vi "MGCC_GetLoadCombinations.vi"(8 "List pf critical loads":dbl[](array[numeric]), 9 "List of loads":dbl[](array[numeric]), 11 "MG topology":dbl[][](array[numeric])) -> (0 "crit_index":i32[](array[numeric]), 1 "ValidComb":i32[][](array[numeric]), 2 "Load_Combinations":i32[][](array[numeric]))   [LabVIEW 2016]
uses:
  <vilib>/imath/engines/lvmath2/RunTimeEngine/IndexRead/NIMS M($,S).vi
  <instcachedir>/0/NIMS M($,S)_3E5749BBB62E49528D4765A77F1F6D98.lvgen/NIMS M($,S)_3E5749BBB62E49528D4765A77F1F6D98_000.vi
  <vilib>/imath/engines/lvmath2/RunTimeEngine/BitwiseOperatorToken/NIMS_Bitwise_Operator_Or.vi
  <instcachedir>/0/NIMS_Bitwise_Operator_Or_51E58CBCE6004B7AAA420A8AC17D98D6.lvgen/NIMS_Bitwise_Operator_Or_51E58CBCE6004B7AAA420A8AC17D98D6_001.vi
  <vilib>/imath/engines/lvmath2/RunTimeEngine/VariableToken/Support/NIMS_Vector Boolean Index to I32 Index.vi
  <vilib>/imath/engines/lvmath2/RunTimeEngine/IndexRead/NIMS M(V,$).vi
  <instcachedir>/0/NIMS M(V,$)_21A5155762F74C04AE4EA67BEE0D3EF5.lvgen/NIMS M(V,$)_21A5155762F74C04AE4EA67BEE0D3EF5_004.vi
  <vilib>/imath/engines/lvmath2/RunTimeEngine/ErrorHandling/NIMS_Create Error From Enums.vi
  <vilib>/imath/engines/lvmath2/RunTimeEngine/BuiltInFunctions/findnz/NIMS_[1o]_findnz(GColV).vi
  <instcachedir>/0/NIMS_[1o]_findnz(GColV)_8556557C9365446B906472366DD9B2D8.lvgen/NIMS_[1o]_findnz(GColV)_8556557C9365446B906472366DD9B2D8_000.vi
  <vilib>/imathl/engines/lvmath/Functions/Error Handling/Create Error.vi
  <vilib>/imath/engines/lvmath2/RunTimeEngine/IndexReplace/NIMS M(V,$)=M.vi
  <instcachedir>/0/NIMS M(V,$)=M_4780607DE7B3494DB49F84B9239A732B.lvgen/NIMS M(V,$)=M_4780607DE7B3494DB49F84B9239A732B_003.vi
  <vilib>/imath/engines/lvmath2/RunTimeEngine/BuiltInFunctions/size/NIMS_I32=size(GM,I32).vi
  <instcachedir>/0/NIMS_I32=size(GM,I32)_122058B1B3294FAEA5DC209B92B394E4.lvgen/NIMS_I32=size(GM,I32)_122058B1B3294FAEA5DC209B92B394E4_004.vi
  <vilib>/imath/engines/lvmath2/RunTimeEngine/BuiltInFunctions/length/NIMS_length(GV).vi
  <instcachedir>/0/NIMS_length(GV)_08A3D13377FD4E4B96F5795FBF3698FA.lvgen/NIMS_length(GV)_08A3D13377FD4E4B96F5795FBF3698FA_000.vi
  <vilib>/imath/engines/lvmath2/RunTimeEngine/RangeToken/NIMS_Range_R2 - Integer.vi
  <instcachedir>/0/NIMS_Range_R2 - Integer_89B873E74E6E489885E44F751DD9C6BF.lvgen/NIMS_Range_R2 - Integer_89B873E74E6E489885E44F751DD9C6BF_000.vi
  <vilib>/imath/engines/lvmath2/RunTimeEngine/CommandStatement/MC_CommandStatement_break.vi
  <vilib>/imath/engines/lvmath2/RunTimeEngine/IndexRead/NIMS V(S).vi
  <instcachedir>/0/NIMS V(S)_0488751826AF41519A22953C041130DC.lvgen/NIMS V(S)_0488751826AF41519A22953C041130DC_000.vi
  <vilib>/imath/engines/lvmath2/RunTimeEngine/IndexReplace/NIMS V(V)=M.vi
  <instcachedir>/0/NIMS V(V)=M_7678915A266E4CDB8C8DB8FB3DB4E364.lvgen/NIMS V(V)=M_7678915A266E4CDB8C8DB8FB3DB4E364_001.vi
  <vilib>/imath/engines/lvmath2/RunTimeEngine/VariableToken/NIMS_VariableToken_CondDefinedDefinedByReplace.vi
  <instcachedir>/0/NIMS_VariableToken_CondDefinedDefinedByReplace_D162CFFC24174562A9FEA619A91E1A56.lvgen/NIMS_VariableToken_CondDefinedDefinedByReplace_D162CFFC24174562A9FEA619A91E1A56_003.vi
  <vilib>/imath/engines/lvmath2/RunTimeEngine/BuiltInFunctions/findnz/NIMS_[1o]_findnz(GRowV).vi
  <instcachedir>/0/NIMS_[1o]_findnz(GRowV)_1AF74843B4874134ADE908C0A4A72F3C.lvgen/NIMS_[1o]_findnz(GRowV)_1AF74843B4874134ADE908C0A4A72F3C_000.vi
  <vilib>/imath/engines/lvmath2/RunTimeEngine/IndexReplace/NIMS V(S)=V.vi
  <instcachedir>/0/NIMS V(S)=V_623363232DF04CF88CEE4AC156064DF2.lvgen/NIMS V(S)=V_623363232DF04CF88CEE4AC156064DF2_000.vi
  <instcachedir>/0/NIMS_VariableToken_CondDefinedDefinedByReplace_D162CFFC24174562A9FEA619A91E1A56.lvgen/NIMS_VariableToken_CondDefinedDefinedByReplace_D162CFFC24174562A9FEA619A91E1A56_002.vi
  <vilib>/imath/engines/lvmath2/RunTimeEngine/IndexRead/NIMS M(S,S).vi
  <instcachedir>/0/NIMS M(S,S)_AC51E74150A542F7991B9634C66F3096.lvgen/NIMS M(S,S)_AC51E74150A542F7991B9634C66F3096_000.vi
  <vilib>/imath/engines/lvmath2/RunTimeEngine/IndexReplace/NIMS M(S,S)=S.vi
  <instcachedir>/0/NIMS M(S,S)=S_98E40400474E4398B113AE20298B4F82.lvgen/NIMS M(S,S)=S_98E40400474E4398B113AE20298B4F82_002.vi
  <vilib>/imath/engines/lvmath2/RunTimeSupport/NIMS_Error if Not Equal.vi
  <instcachedir>/0/NIMS_Error if Not Equal_43252A79AD05436189442EC0C5E5AB8A.lvgen/NIMS_Error if Not Equal_43252A79AD05436189442EC0C5E5AB8A_000.vi
  <vilib>/imath/engines/lvmath2/RunTimeEngine/VariableToken/NIMS_VariableToken_CondDefined.vi
  <instcachedir>/0/NIMS_VariableToken_CondDefined_06E9DA95BD4D46A6BA55EC651A891960.lvgen/NIMS_VariableToken_CondDefined_06E9DA95BD4D46A6BA55EC651A891960_009.vi
  <instcachedir>/0/NIMS_I32=size(GM,I32)_122058B1B3294FAEA5DC209B92B394E4.lvgen/NIMS_I32=size(GM,I32)_122058B1B3294FAEA5DC209B92B394E4_005.vi
  <instcachedir>/0/NIMS_VariableToken_CondDefined_06E9DA95BD4D46A6BA55EC651A891960.lvgen/NIMS_VariableToken_CondDefined_06E9DA95BD4D46A6BA55EC651A891960_005.vi
  <vilib>/imath/engines/lvmath2/RunTimeEngine/BuiltInFunctions/zeros/NIMS_V=zeros(I32,I32).vi
  <vilib>/imath/engines/lvmath2/RunTimeEngine/IndexReplace/NIMS V(V)=S.vi
  <instcachedir>/0/NIMS V(V)=S_4469BB7E0DD5440190F262393D16598E.lvgen/NIMS V(V)=S_4469BB7E0DD5440190F262393D16598E_001.vi
  <instcachedir>/0/NIMS_Error if Not Equal_43252A79AD05436189442EC0C5E5AB8A.lvgen/NIMS_Error if Not Equal_43252A79AD05436189442EC0C5E5AB8A_001.vi
  <vilib>/imath/engines/lvmath2/RunTimeEngine/IndexReplace/NIMS V(S)=S.vi
  <instcachedir>/0/NIMS V(S)=S_57E16554CB8B4B90AAB163894F717546.lvgen/NIMS V(S)=S_57E16554CB8B4B90AAB163894F717546_003.vi
  <vilib>/imath/engines/lvmath2/RunTimeEngine/BuiltInFunctions/ones/NIMS_V=ones(I32,I32).vi
  <vilib>/imath/engines/lvmath2/RunTimeEngine/RowToken/NIMS_RowToken_M_M.vi
  <instcachedir>/0/NIMS_RowToken_M_M_968CDE3545E74ACDAEA4B48DE01EEECA.lvgen/NIMS_RowToken_M_M_968CDE3545E74ACDAEA4B48DE01EEECA_005.vi
  <vilib>/imath/engines/lvmath2/RunTimeEngine/MatrixToken/NIMS_MatrixToken_M_M.vi
  <instcachedir>/0/NIMS_MatrixToken_M_M_DF273B0CC20F424BBF1EDA9F4E71C841.lvgen/NIMS_MatrixToken_M_M_DF273B0CC20F424BBF1EDA9F4E71C841_005.vi
  <vilib>/imath/engines/lvmath2/RunTimeEngine/BuiltInFunctions/fmin_lp/NIMS_fmin_lp.vi
  <instcachedir>/0/NIMS_VariableToken_CondDefinedDefinedByReplace_D162CFFC24174562A9FEA619A91E1A56.lvgen/NIMS_VariableToken_CondDefinedDefinedByReplace_D162CFFC24174562A9FEA619A91E1A56_001.vi
  <vilib>/imath/engines/lvmath2/RunTimeEngine/IndexRead/NIMS V(R2).vi
  <instcachedir>/0/NIMS V(R2)_C76619605A0E4E9F8B2FA9389712AC47.lvgen/NIMS V(R2)_C76619605A0E4E9F8B2FA9389712AC47_000.vi
  <vilib>/imath/engines/lvmath2/RunTimeEngine/ArithmeticOperatorToken/NIMS_ArithmeticOperator_minus.vi
  <instcachedir>/0/NIMS_ArithmeticOperator_minus_E3B65B1D26A44BB184AFDC5B3F458E3D.lvgen/NIMS_ArithmeticOperator_minus_E3B65B1D26A44BB184AFDC5B3F458E3D_003.vi
  <vilib>/imath/engines/lvmath2/RunTimeEngine/IndexReplace/NIMS M($,S)=V.vi
  <instcachedir>/0/NIMS M($,S)=V_EEA74323A7E5479BB387BE0F93352290.lvgen/NIMS M($,S)=V_EEA74323A7E5479BB387BE0F93352290_001.vi
  <instcachedir>/0/NIMS_VariableToken_CondDefined_06E9DA95BD4D46A6BA55EC651A891960.lvgen/NIMS_VariableToken_CondDefined_06E9DA95BD4D46A6BA55EC651A891960_001.vi
  <vilib>/imath/engines/lvmath2/RunTimeEngine/BuiltInFunctions/abs/NIMS_abs(signed).vi
  <instcachedir>/0/NIMS_abs(signed)_C4FCB8E6058B49B797C7C8D53CA5F6EC.lvgen/NIMS_abs(signed)_C4FCB8E6058B49B797C7C8D53CA5F6EC_005.vi
  <vilib>/imath/engines/lvmath2/RunTimeEngine/VariableToken/Support/NIMS_Matrix Boolean Index to I32 Index.vi
  <vilib>/imath/engines/lvmath2/RunTimeEngine/IndexReplace/NIMS M(V)=S.vi
  <instcachedir>/0/NIMS M(V)=S_F2304187E1344F60ABCBE5C5CC0920F9.lvgen/NIMS M(V)=S_F2304187E1344F60ABCBE5C5CC0920F9_000.vi
  <instcachedir>/0/NIMS_length(GV)_08A3D13377FD4E4B96F5795FBF3698FA.lvgen/NIMS_length(GV)_08A3D13377FD4E4B96F5795FBF3698FA_002.vi
  <vilib>/imath/engines/lvmath2/RunTimeEngine/RangeToken/NIMS_Range.vi
  <instcachedir>/0/NIMS_Range_A7C094595B484CA7AF10685B02D808ED.lvgen/NIMS_Range_A7C094595B484CA7AF10685B02D808ED_001.vi
  <vilib>/imath/engines/lvmath/Functions/Error Handling/MergeErrorsWrapper.vi
  <vilib>/imath/engines/lvmath2/RunTimeEngine/NodeEndStatement/NIMS_NodeEndStatement_Output.vi
  <instcachedir>/0/NIMS_NodeEndStatement_Output_53EC0D466D134D7ABD903AC30B43404B.lvgen/NIMS_NodeEndStatement_Output_53EC0D466D134D7ABD903AC30B43404B_004.vi
  <instcachedir>/0/NIMS_NodeEndStatement_Output_53EC0D466D134D7ABD903AC30B43404B.lvgen/NIMS_NodeEndStatement_Output_53EC0D466D134D7ABD903AC30B43404B_005.vi
  <instcachedir>/0/NIMS_NodeEndStatement_Output_53EC0D466D134D7ABD903AC30B43404B.lvgen/NIMS_NodeEndStatement_Output_53EC0D466D134D7ABD903AC30B43404B_011.vi
  <instcachedir>/0/NIMS_NodeEndStatement_Output_53EC0D466D134D7ABD903AC30B43404B.lvgen/NIMS_NodeEndStatement_Output_53EC0D466D134D7ABD903AC30B43404B_002.vi
  <vilib>/imath/engines/lvmath2/RunTimeEngine/ErrorHandling/NIMS_Finalize Error.vi
  <vilib>/Analysis/Matrix/Numeric/Conversions/Matrix To Array - RM.vi
  <vilib>/imath/engines/lvmath2/RunTimeEngine/BuiltInFunctions/size/NIMS_[I32,I32]=size(GM).vi
  <instcachedir>/0/NIMS_[I32,I32]=size(GM)_B0A6EC1255BB4C8AB801FE6F734128D9.lvgen/NIMS_[I32,I32]=size(GM)_B0A6EC1255BB4C8AB801FE6F734128D9_000.vi
  <vilib>/imath/engines/lvmath2/RunTimeEngine/MatrixToken/NIMS_MatrixToken_M_RV.vi
  <instcachedir>/0/NIMS_MatrixToken_M_RV_EE14907D4B194E829889005D2F556E9C.lvgen/NIMS_MatrixToken_M_RV_EE14907D4B194E829889005D2F556E9C_002.vi
  <instcachedir>/0/NIMS_NodeEndStatement_Output_53EC0D466D134D7ABD903AC30B43404B.lvgen/NIMS_NodeEndStatement_Output_53EC0D466D134D7ABD903AC30B43404B_010.vi
  <instcachedir>/0/NIMS_[I32,I32]=size(GM)_B0A6EC1255BB4C8AB801FE6F734128D9.lvgen/NIMS_[I32,I32]=size(GM)_B0A6EC1255BB4C8AB801FE6F734128D9_005.vi
  <vilib>/imath/engines/lvmath2/RunTimeEngine/IndexRead/NIMS M($,R2).vi
  <instcachedir>/0/NIMS M($,R2)_D9380E19261A4ADFB2D364AF6959C6EF.lvgen/NIMS M($,R2)_D9380E19261A4ADFB2D364AF6959C6EF_001.vi
  <vilib>/imath/engines/lvmath2/RunTimeEngine/IndexRead/NIMS M(S,$).vi
  <instcachedir>/0/NIMS M(S,$)_F24F360562DE41D8BE234322A2E15C65.lvgen/NIMS M(S,$)_F24F360562DE41D8BE234322A2E15C65_002.vi
  <vilib>/imath/engines/lvmath2/RunTimeEngine/BuiltInFunctions/sum/NIMS_sum(GV).vi
  <instcachedir>/0/NIMS_sum(GV)_67F5EC36BC034E54A6BEC5B0673C00E5.lvgen/NIMS_sum(GV)_67F5EC36BC034E54A6BEC5B0673C00E5_000.vi
  <vilib>/imath/engines/lvmath2/RunTimeEngine/BuiltInFunctions/findnz/NIMS_[1o]_findnz(GM).vi
  <instcachedir>/0/NIMS_[1o]_findnz(GM)_0B85F0C1FD7A4D70A7D15487030BA0C8.lvgen/NIMS_[1o]_findnz(GM)_0B85F0C1FD7A4D70A7D15487030BA0C8_003.vi
  <vilib>/imath/engines/lvmath2/RunTimeEngine/BuiltInFunctions/is_empty/NIMS_is_empty(GM).vi
  <instcachedir>/0/NIMS_is_empty(GM)_AF8F13F4B7FD436CB1855477E2504B8A.lvgen/NIMS_is_empty(GM)_AF8F13F4B7FD436CB1855477E2504B8A_005.vi
  <vilib>/imath/engines/lvmath2/RunTimeEngine/IndexRead/NIMS M(S,V).vi
  <instcachedir>/0/NIMS M(S,V)_5C1965D37F59432CA0E9661793EAFE90.lvgen/NIMS M(S,V)_5C1965D37F59432CA0E9661793EAFE90_001.vi
  <vilib>/imath/engines/lvmath2/RunTimeEngine/BuiltInFunctions/sets_unique/NIMS_sets_unique(GM).vi
  <instcachedir>/0/NIMS_sets_unique(GM)_A55EFC7C1FC44AA39E21562D64C6E0C8.lvgen/NIMS_sets_unique(GM)_A55EFC7C1FC44AA39E21562D64C6E0C8_002.vi
  <vilib>/imath/engines/lvmath2/RunTimeEngine/BuiltInFunctions/length/NIMS_length(GM).vi
  <instcachedir>/0/NIMS_length(GM)_47CEC356FCE0482D9BA47DC61C99F2C7.lvgen/NIMS_length(GM)_47CEC356FCE0482D9BA47DC61C99F2C7_000.vi
  <vilib>/imath/engines/lvmath2/RunTimeEngine/IndexRead/NIMS M(S).vi
  <instcachedir>/0/NIMS M(S)_B826C018497E4940AE96BD27B540B6FB.lvgen/NIMS M(S)_B826C018497E4940AE96BD27B540B6FB_000.vi
  <vilib>/imath/engines/lvmath2/RunTimeEngine/IndexRead/NIMS V(V).vi
  <instcachedir>/0/NIMS V(V)_298D9CB7BFEB42B8BC8D9C3C28AE8C70.lvgen/NIMS V(V)_298D9CB7BFEB42B8BC8D9C3C28AE8C70_001.vi
  <vilib>/imath/engines/lvmath2/RunTimeEngine/MatrixToken/NIMS_MatrixToken_M_SorCV.vi
  <instcachedir>/0/NIMS_MatrixToken_M_SorCV_D3266533510A4291A747E91CF193467A.lvgen/NIMS_MatrixToken_M_SorCV_D3266533510A4291A747E91CF193467A_003.vi
  <vilib>/imath/engines/lvmath2/RunTimeEngine/IndexReplace/NIMS M(M,$)=M.vi
  <instcachedir>/0/NIMS M(M,$)=M_DC36964DDF7C4131B957B72D426BDC22.lvgen/NIMS M(M,$)=M_DC36964DDF7C4131B957B72D426BDC22_003.vi
  <vilib>/Analysis/Matrix/NI_Matrix.lvlib
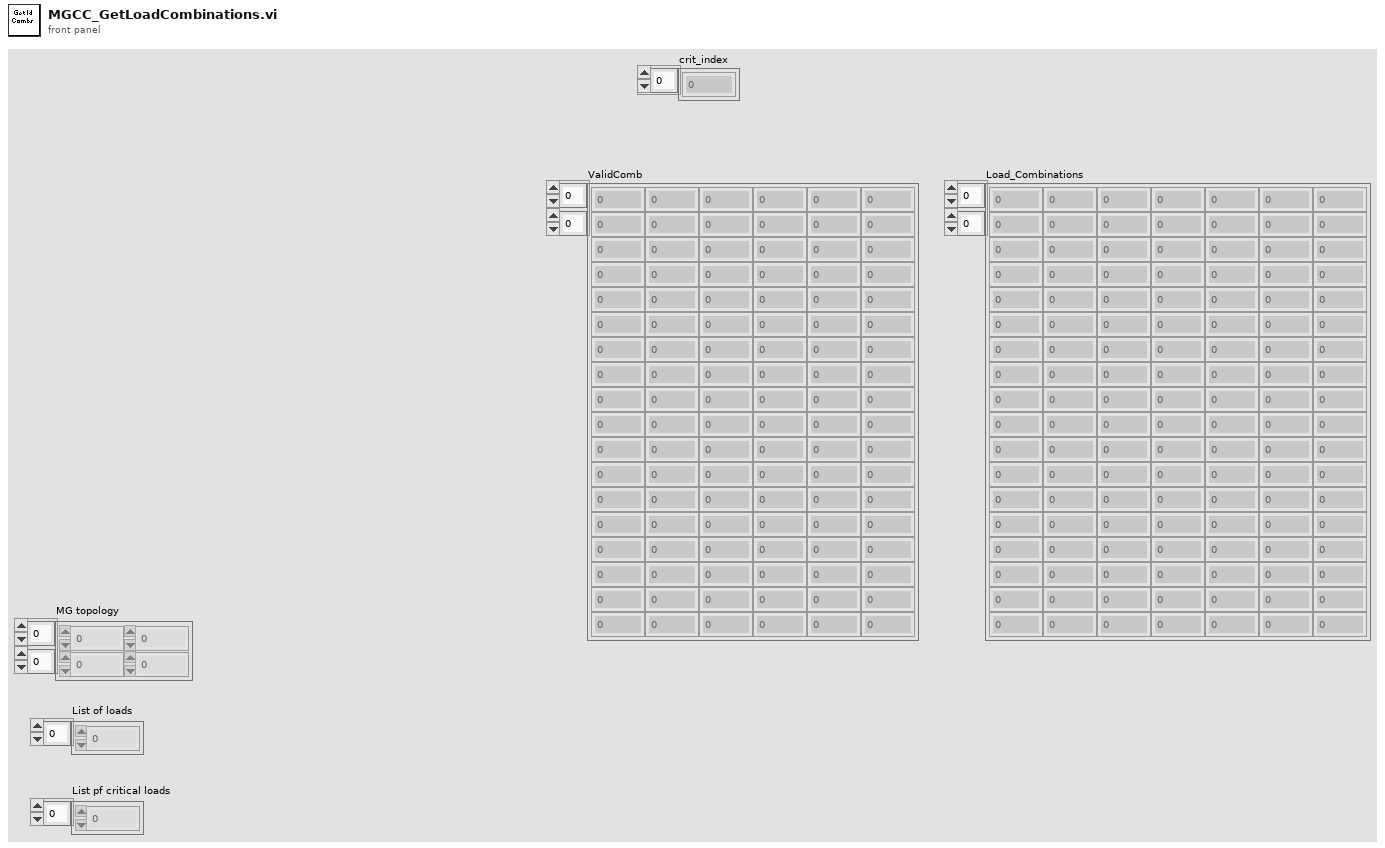
[diagram p1: front panel]
types:
  T1 = typedef "NI_Matrix.lvlib/RealMatrix.ctl" = dbl[][]
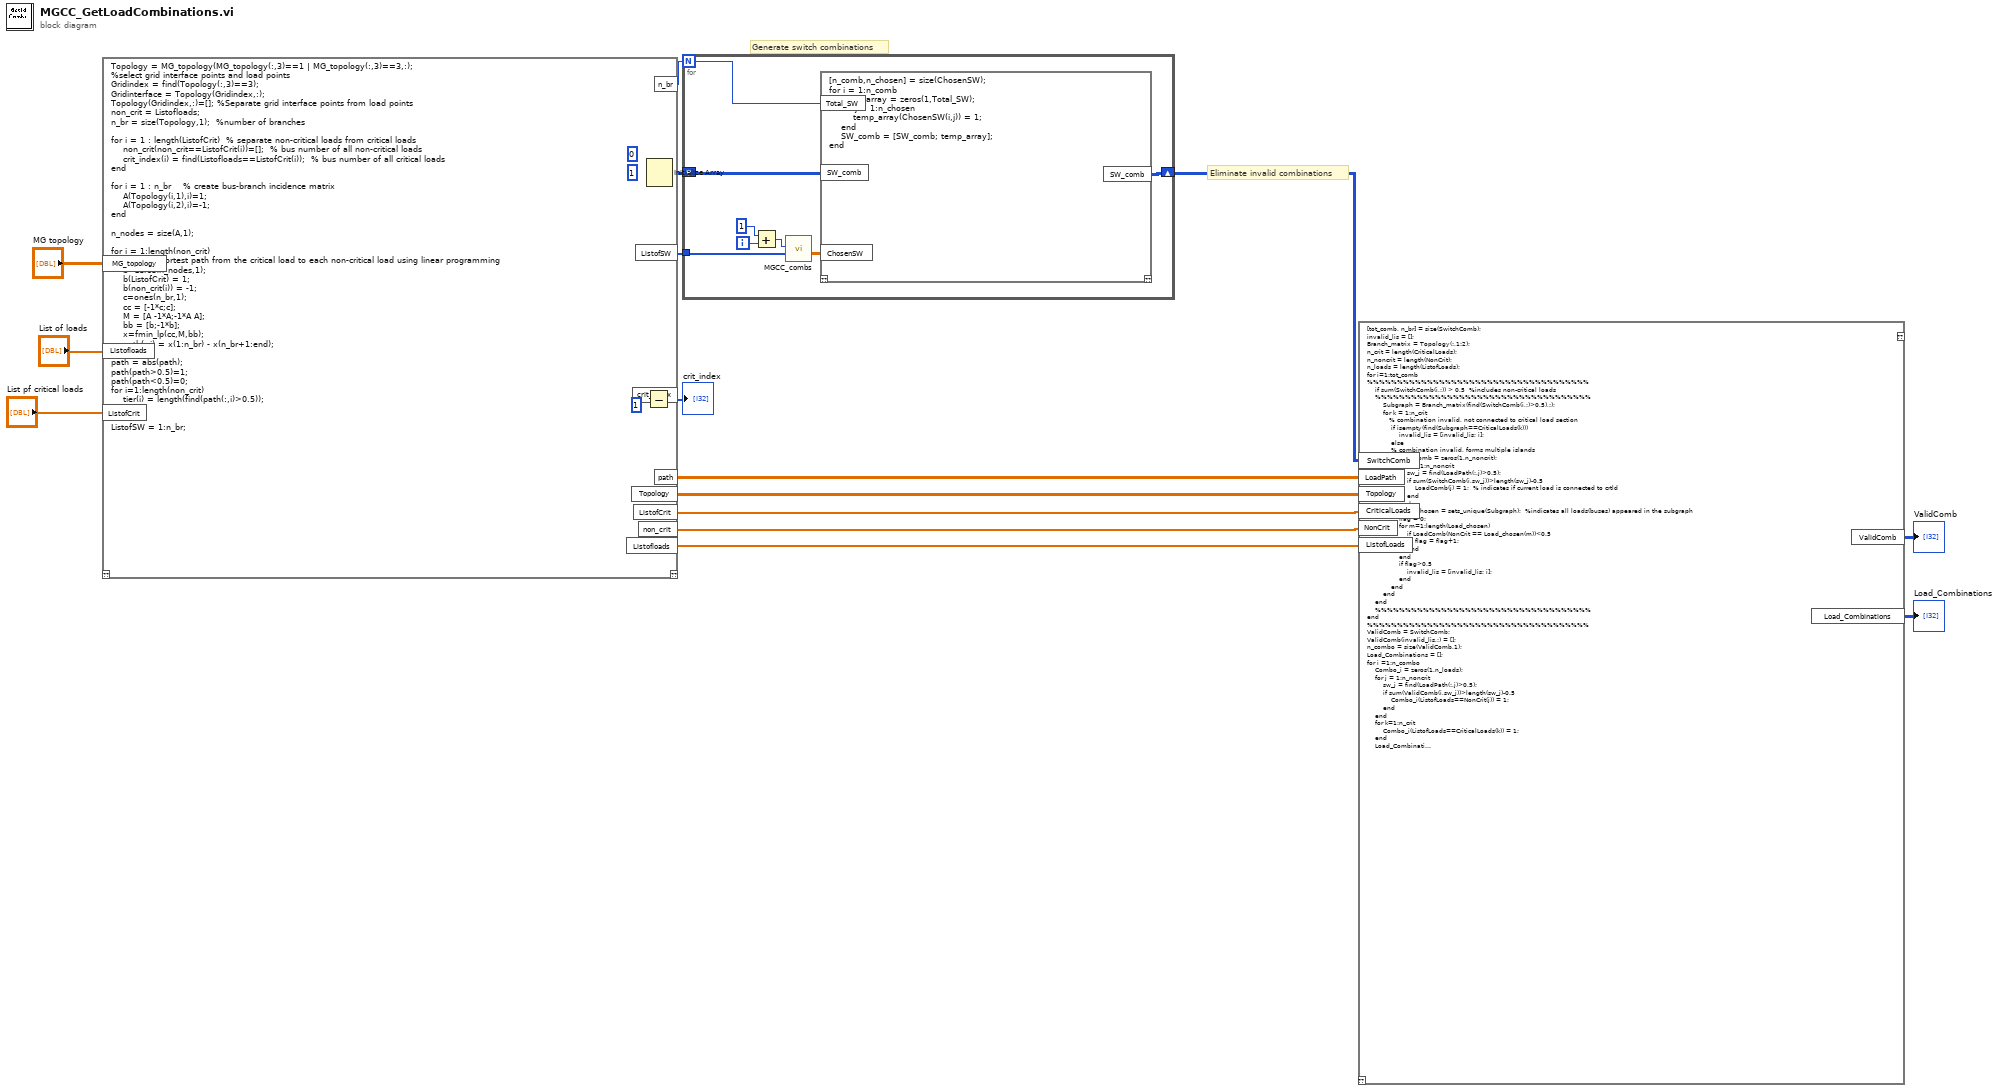
[diagram p0: block diagram]
diagram:
  # "Eliminate invalid combinations"
  # "Generate switch combinations"
  n1 = mathscript code="Topology = MG_topology(MG_topology(:,3)==1 | MG_topology(:,3)==3,:);  \n%select grid interface points and load points\nGridindex = find(Topology(:,3)==3);\nGridinterface = Topology(Gridindex,:);\nTopology(Gridindex,:)=[]; %Separate grid interface points from load points\nnon_crit = Listofloads;\nn_br = size(Topology,1);  %number of branches\n\nfor i = 1 : length(ListofCrit)  % separate non-critical loads from critical loads\n    non_crit(non_crit==ListofCrit(i))=[];  % bus number of all non-critical loads\n    crit_index(i) = find(Listofloads==ListofCrit(i));  % bus number of all critical loads\nend\n\nfor i = 1 : n_br    % create bus-branch incidence matrix\n    A(Topology(i,1),i)=1;\n    A(Topology(i,2),i)=-1;\nend\n\nn_nodes = size(A,1);\n\nfor i = 1:length(non_crit)   \n% find the shortest path from the critical load to each non-critical load using linear programming\n    b=zeros(n_nodes,1);\n    b(ListofCrit) = 1;\n    b(non_crit(i)) = -1;\n    c=ones(n_br,1);\n    cc = [-1*c;c];\n    M = [A -1*A;-1*A A];\n    bb = [b;-1*b];\n    x=fmin_lp(cc,M,bb);\n    path(:,i) = x(1:n_br) - x(n_br+1:end);\nend\npath = abs(path);\npath(path>0.5)=1;\npath(path<0.5)=0;\nfor i=1:length(non_crit)\n    tier(i) = length(find(path(:,i)>0.5));\nend\n\nListofSW = 1:n_br;"("MG_topology"="MG topology", "Listofloads"="List of loads", "ListofCrit"="List pf critical loads") -> ("Topology"=w7:dbl[][], "non_crit"=w6:dbl[], "path"=w8:dbl[][], "ListofSW"=w12:i32[], "n_br"=w14:i32, "ListofCrit"=w5:dbl[], "Listofloads"=w4:dbl[], "crit_index"=w3:i32[])  [unwired: 1 in, 1 out]
  n2 = Subtract(x=w3, y=1) -> (x-y=→"crit_index":i32[])
  n3 = Initialize Array(0 ("element"), 1 ("dimension size"), w14) -> (w13:i32[][])
  n4 = for {
    N: w14 -> [w25]
    tunnel: w12 -> [w21]
    shift-right: [w23] -> w9
    shift-left: w13 -> [w24]
    i -> [w27]
    n5 = Add(x=1, y=w27) -> (x+y=w22:i32)
    n6 = call "MGCC_combs.vi"("v"=w21, "m"=w22) -> ("P"=w20:T1)  [unwired: 9 in]
    n7 = mathscript code="[n_comb,n_chosen] = size(ChosenSW);\nfor i = 1:n_comb\n    temp_array = zeros(1,Total_SW);\n    for j = 1:n_chosen\n        temp_array(ChosenSW(i,j)) = 1;\n    end\n    SW_comb = [SW_comb; temp_array];\nend"("ChosenSW"=w20, "Total_SW"=w25, "SW_comb"=w24) -> ("SW_comb"=w23:i32[][])  [unwired: 1 in, 1 out]
  }
  n8 = mathscript code="[tot_comb, n_br] = size(SwitchComb);\ninvalid_lis = [];\nBranch_matrix = Topology(:,1:2);\nn_crit = length(CriticalLoads);\nn_noncrit = length(NonCrit);\nn_loads = length(ListofLoads);\nfor i=1:tot_comb\n%%%%%%%%%%%%%%%%%%%%%%%%%%%%%%%%%%%%%\n    if sum(SwitchComb(i,:)) > 0.5  %includes non-critical loads\n    %%%%%%%%%%%%%%%%%%%%%%%%%%%%%%%%%%%%\n        Subgraph = Branch_matrix(find(SwitchComb(i,:)>0.5),:);\n        for k = 1:n_crit\n           % combination invalid, not connected to critical load section\n            if isempty(find(Subgraph==CriticalLoads(k)))   \n                invalid_lis = [invalid_lis; i];\n            else\n            % combination invalid, forms multiple islands\n                LoadComb = zeros(1,n_noncrit);\n                for j = 1:n_noncrit\n                    sw_j = find(LoadPath(:,j)>0.5);\n                    if sum(SwitchComb(i,sw_j))>length(sw_j)-0.5\n                        LoadComb(j) = 1;  % indicates if current load is connected to crtld\n                    end\n                end\n                Load_chosen = sets_unique(Subgraph);  %indicates all loads(buses) appeared in the subgraph\n                flag = 0;\n                for m=1:length(Load_chosen)\n                    if LoadComb(NonCrit == Load_chosen(m))<0.5\n                        flag = flag+1;\n                    end\n                end\n                if flag>0.5\n                    invalid_lis = [invalid_lis; i];\n                end\n            end\n        end\n    end\n    %%%%%%%%%%%%%%%%%%%%%%%%%%%%%%%%%%%%\nend\n%%%%%%%%%%%%%%%%%%%%%%%%%%%%%%%%%%%%%\nValidComb = SwitchComb;\nValidComb(invalid_lis,:) = [];\nn_combo = size(ValidComb,1);\nLoad_Combinations = [];\nfor i =1:n_combo\n    Combo_i = zeros(1,n_loads);\n    for j = 1:n_noncrit\n        sw_j = find(LoadPath(:,j)>0.5);\n        if sum(ValidComb(i,sw_j))>length(sw_j)-0.5\n            Combo_i(ListofLoads==NonCrit(j)) = 1;\n        end\n    end\n    for k=1:n_crit\n        Combo_i(ListofLoads==CriticalLoads(k)) = 1;\n    end\n    Load_Combinations = [Load_Combinations; Combo_i];\nend"("SwitchComb"=w9, "Topology"=w7, "LoadPath"=w8, "CriticalLoads"=w5, "NonCrit"=w6, "ListofLoads"=w4) -> ("ValidComb"=→"ValidComb":i32[][], "Load_Combinations"=→"Load_Combinations":i32[][])  [unwired: 1 in, 1 out]
